vi "publishGrating.vi"(8 "error in (no error)":errorcluster, 10 "GratingType":T1=enum."Red", 11 "MonoCommunicator in":refnum<class "MonoCommunicator.lvclass">) -> (0 "error out":errorcluster, 3 "MonoCommunicator out":refnum<class "MonoCommunicator.lvclass">)   [LabVIEW 2016, in "MonoCommunicator.lvclass"]
uses:
  MonoCommunicator.lvclass
  Typedefs/GratingType.ctl
  Typedefs/publishers.ctl
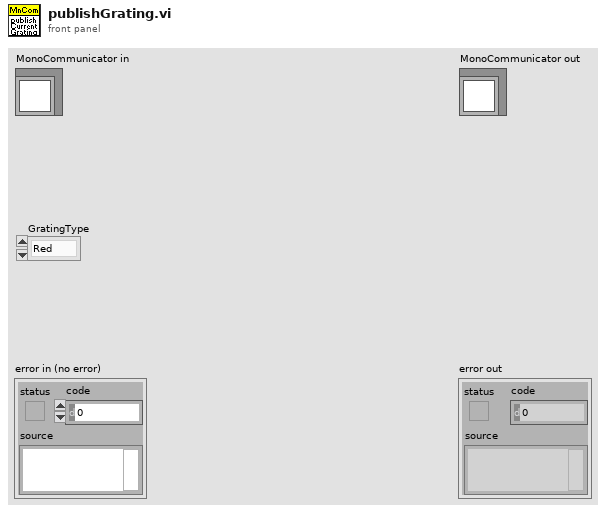
[diagram p1: front panel]
types:
  T1 = typedef "GratingType.ctl" = enum16{"Blue", "Red", "Mirror"}
  T2 = typedef "publishers.ctl" = enum16{"Wavelength", "Grating", "FrontEntranceSlitPosition", "FrontExitSlitPosition", "SoftwareStatus", "MonochromatorId", "Ack"}
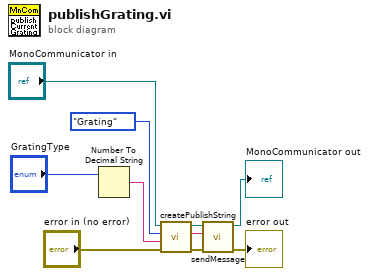
[diagram p0: block diagram]
diagram:
  n1 = Number To Decimal String(number="GratingType") -> (decimal integer string=w1:string)  [unwired: 1 in]
  n2 = call "createPublishString.vi"("error in (no error)"="error in (no error)", "parameter"=w1, "publishers"=publishers."Grating", "MonoCommunicator in"="MonoCommunicator in") -> ("error out"=w6:errorcluster, "string"=w4:string, "MonoCommunicator out"=w5:refnum<class "MonoCommunicator.lvclass">)  [unwired: 5 in]
  n3 = call-dynamic "sendMessage.vi"("error in (no error)"=w6, "message"=w4, "MonoCommunicator in"=w5) -> ("error out"=→"error out":errorcluster, "MonoCommunicator out"=→"MonoCommunicator out":refnum<class "MonoCommunicator.lvclass">)  [unwired: 7 in]
